vi "Main_08b refactored.vi"() -> ()   [LabVIEW 2020]
panel:
  out "max value":i32
  out "Puzzle Array":i32[][](array[numeric])
  in  "Puzzle":string="200200221023111313131033314121142013103432145142351212334232423210101340410243413011333312111010010\n021002023301222221234134021422342024344555521535143232341414552024224120114233210330203002020100112\n120000123021210023111321143114331115334535223455511513445233523154411102203411040133312002213001021\n110211312303200204232110124204135453554533435152342542252215415141133330323032234114310011301232202\n112002122201001100330432244432552555524445123151222142521452233321152332132412434434431321322021220\n000131233030332102140440124221314455255431113413445553414144524134315351524134030112312012102102122\n..."
  in  "Example":string="30373\n25512\n65332\n33549\n35390"
  # "--- Part Two ---\nContent with the amount of tree cover available, the Elves just need to know the best spot to build their tree house: they would like to be able to see a lot of trees.\n\nTo measure the viewing distance from a given tree, look up, down, left, and right from that tree; stop if you reach an edge or at the first tree that is the same height or taller than the tree under consideration. (If a tree is right on the edge, at least one of its viewing distances will be zero.)\n\nThe Elves don't care about distant trees taller than those found by the rules above; the proposed tree house has large eaves to keep it dry, so they wouldn't be able to see higher than the tree house anyway.\n\nIn the example above, consider the middle 5 in the second row:\n\n30373\n25512\n65332\n33549\n35390\nLooking up, its view is not blocked; it can see 1 tree (of height 3).\nLooking left, its view is blocked immediately; it can see only 1 tree (of height 5, right next to it).\nLooking right, its view is not blocked; it can see 2 trees.\nLooking down, its view is blocked eventually; it can see 2 trees (one of height 3, then the tree of height 5 that blocks its view).\nA tree's scenic score is found by multiplying together its viewing distance in each of the four directions. For this tree, this is 4 (found by multiplying 1 * 1 * 2 * 2).\n\nHowever, you can do even better: consider the tree of height 5 in the middle of the fourth row:\n\n30373\n25512\n65332\n33549\n35390\nLooking up, its view is blocked at 2 trees (by another tree with a height of 5).\nLooking left, its view is not blocked; it can see 2 trees.\nLooking down, its view is also not blocked; it can see 1 tree.\nLooking right, its view is blocked at 2 trees (by a massive tree of height 9).\nThis tree's scenic score is 8 (2 * 2 * 1 * 2); this is the ideal spot for the tree house.\n\nConsider each tree on your map. What is the highest scenic score possible for any tree?"
  # "368368."
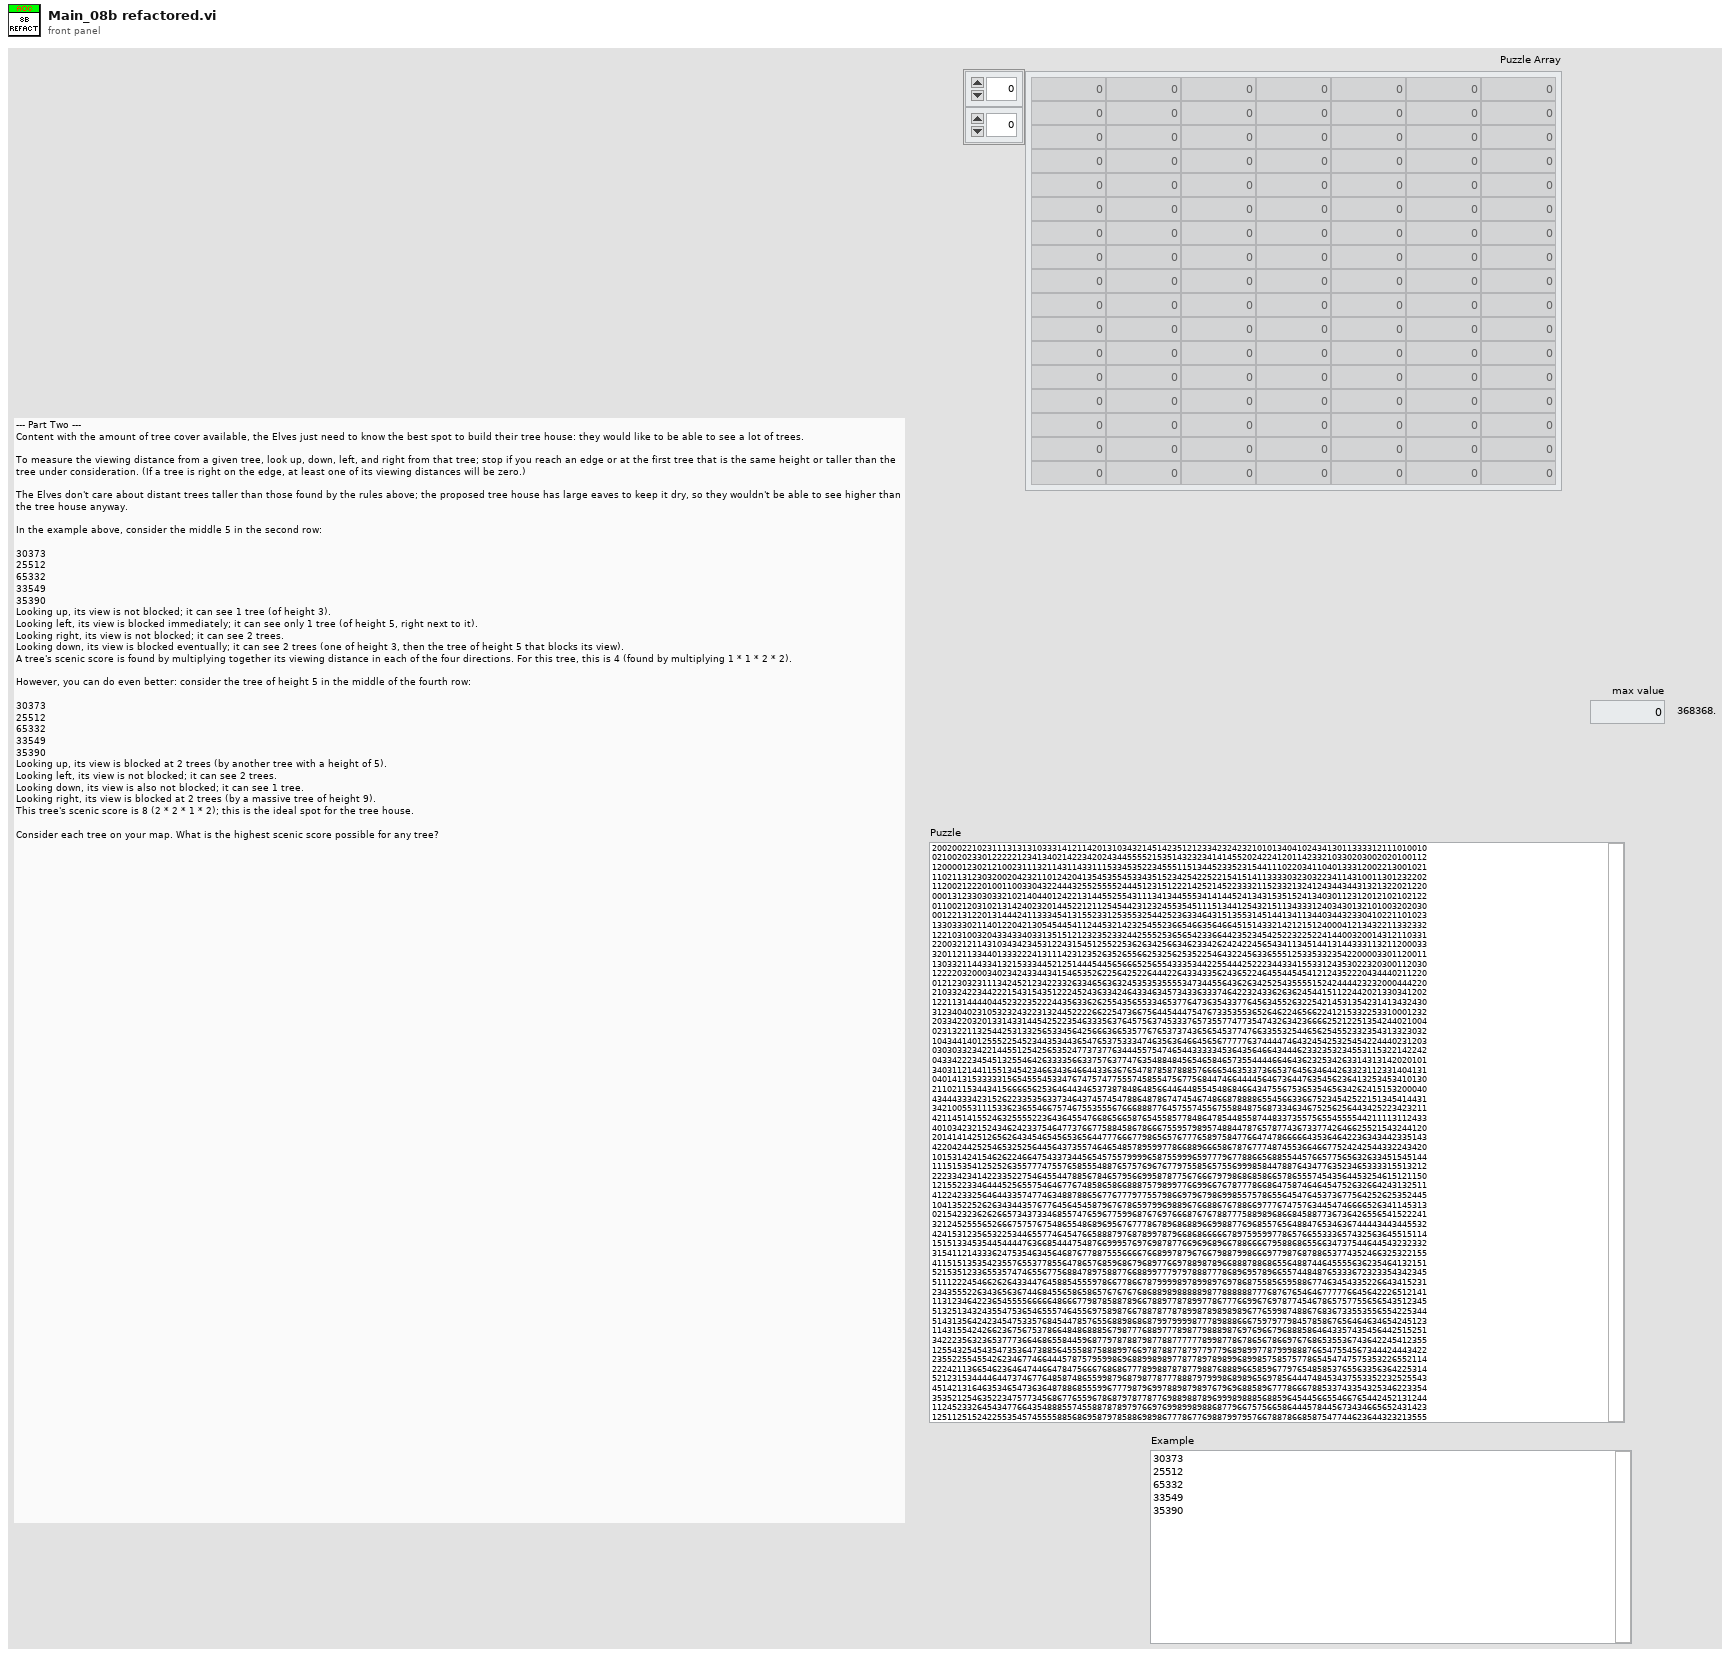
[diagram p1: front panel]
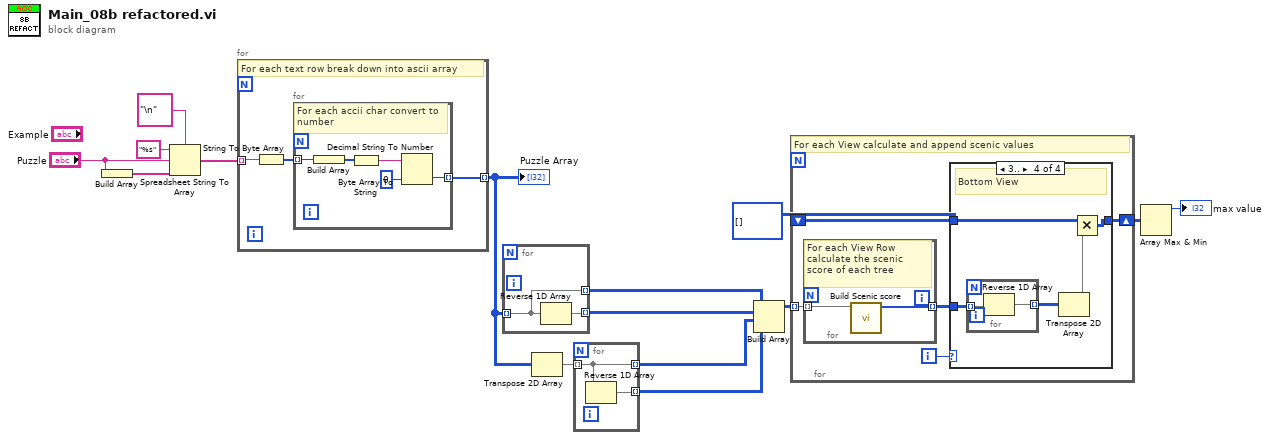
[diagram p0: block diagram]
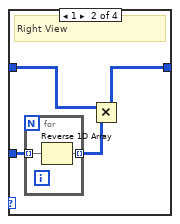
[diagram p3: hidden frame]
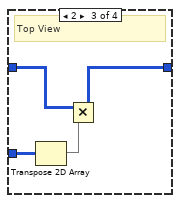
[diagram p4: hidden frame]
diagram:
  n1 = Build Array("Puzzle") -> (w15:string[])
  n2 = Spreadsheet String To Array(delimiter (Tab)="\n", format string="%s", spreadsheet string="Puzzle", array type (2D Dbl)=w15) -> (array=w12:string[])
  n3 = for {
    tunnel: w12 -> [w18] mode=indexing
    tunnel: [w16] -> w10 mode=indexing
    # "For each text row break down into ascii array"
    n4 = String To Byte Array(string=w18) -> (unsigned byte array=w17:u8[])
    n5 = for {
      tunnel: w17 -> [w23] mode=indexing
      tunnel: [w19] -> w16 mode=indexing
      # "For each accii char convert to number"
      n6 = Build Array(w23) -> (w22:u8[])
      n7 = Byte Array To String(unsigned byte array=w22) -> (string=w21:string)
      n8 = Decimal String To Number(string=w21, default (0L)=0 ("default (0 I32)")) -> (number=w19:i32)  [unwired: 1 in, 1 out]
    }
  }
  "Puzzle Array" <- w10
  n9 = for {
    tunnel: w10 -> [w24] mode=indexing
    tunnel: [w25] -> w7 mode=indexing
    tunnel: [w24] -> w8 mode=indexing
    n10 = Reverse 1D Array(array=w24) -> (reversed array=w25:i32[])
  }
  n11 = Transpose 2D Array(2D array=w10) -> (transposed array=w9:i32[][])
  n12 = for {
    tunnel: w9 -> [w26] mode=indexing
    tunnel: [w27] -> w5 mode=indexing
    tunnel: [w26] -> w6 mode=indexing
    n13 = Reverse 1D Array(array=w26) -> (reversed array=w27:i32[])
  }
  n14 = Build Array(w8, w7, w6, w5) -> (w11:i32[][][])
  n15 = for {
    tunnel: w11 -> [w32] mode=indexing
    shift-right: [w28] -> w3
    shift-left: i32[][] [] -> [w29]
    i -> [w30]
    # "For each View calculate and append scenic values"
    n16 = for {
      tunnel: w32 -> [w33] mode=indexing
      tunnel: [w34] -> w31 mode=indexing
      # "For each View Row calculate the scenic score of each tree"
      n17 = call "Build Scenic score.vi"("Array in"=w33) -> ("Secinic score"=w34:i32[])  [unwired: 10 in]
    }
    n18 = case shown="3.." w30 {
      tunnel: w31 -> [w35 w39 w45 w50]
      tunnel: w29 -> [_ w38 w44 w48]
      tunnel: [w35 w36 w42 w47] -> w28
      frame ..0 {
        # "Left View"
      }
      frame 1 {
        # "Right View"
        n19 = for {
          tunnel: w39 -> [w41] mode=indexing
          tunnel: [w40] -> w37 mode=indexing
          n20 = Reverse 1D Array(array=w41) -> (reversed array=w40:i32[])
        }
        n21 = Multiply(x=w38, y=w37) -> (x*y=w36:i32[][])
      }
      frame 2 {
        # "Top View"
        n22 = Transpose 2D Array(2D array=w45) -> (transposed array=w43:i32[][])
        n23 = Multiply(x=w44, y=w43) -> (x*y=w42:i32[][])
      }
      frame 3.. {
        # "Bottom View"
        n24 = for {
          tunnel: w50 -> [w52] mode=indexing
          tunnel: [w51] -> w49 mode=indexing
          n25 = Reverse 1D Array(array=w52) -> (reversed array=w51:i32[])
        }
        n26 = Transpose 2D Array(2D array=w49) -> (transposed array=w46:i32[][])
        n27 = Multiply(x=w48, y=w46) -> (x*y=w47:i32[][])
      }
    }
  }
  n28 = Array Max & Min(array=w3) -> (max value=→"max value":i32)  [unwired: 3 out]
